vi "AIV.vi"() -> ()   [LabVIEW 2014]
uses:
  <vilib>/Rock Robotics/WPI/SerialPort/WPI_SerialPort.ctl
panel:
  out "all currents (A)":dbl[](array[numeric])
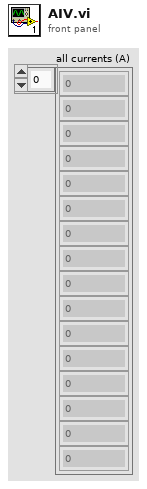
[diagram p1: front panel]
types:
  T1 = typedef "WPI_SerialPort.ctl" = enum16{"Onboard RS-232", "MXP TTL"}
  T2 = typedef "WPI_SerialPortRef.ctl" = cluster{"DevStatus":errorcluster, "Serial Port Name":refnum<visa-resource-name>}
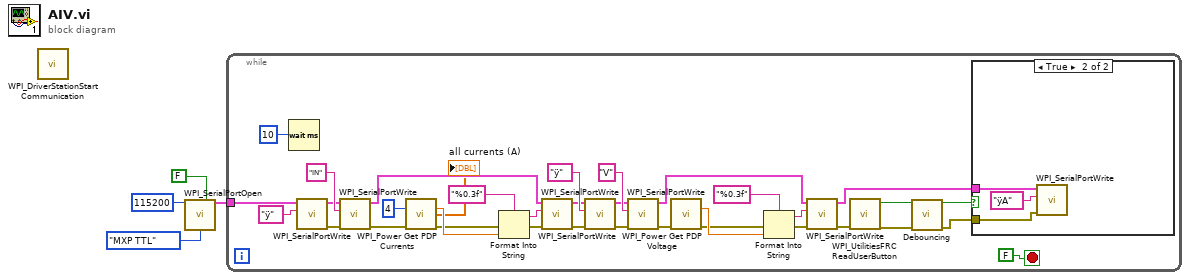
[diagram p0: block diagram]
diagram:
  n1 = call <vilib>:"WPI_DriverStationStart Communication.vi"() -> ()  [unwired: 12 in]
  n2 = call <vilib>:"WPI_SerialPortOpen.vi"("Baud Rate"=u32 115200, "Enable Termination Char? (T)"=FALSE, "Serial Port"=WPI_SerialPort."MXP TTL") -> ("SerialPortRef"=w3:T2)  [unwired: 11 in, 1 out]
  n3 = while {
    tunnel: w3 -> [w36]
    stop <- FALSE stop-if-true
    n4 = Wait (ms)(milliseconds to wait=u32 10) -> ()  [unwired: 1 out]
    n5 = call <vilib>:"WPI_SerialPortWrite.vi"("Buffer"="ÿ", "SerialPortRef"=w36) -> ("error out"=w29:errorcluster, "SerialPortRef"=w30:T2)  [unwired: 7 in, 1 out]
    n6 = call <vilib>:"WPI_SerialPortWrite.vi"("error in (no error)"=w29, "Buffer"="IN", "SerialPortRef"=w30) -> ("error out"=w32:errorcluster, "SerialPortRef"=w25:T2)  [unwired: 6 in, 1 out]
    n7 = call <vilib>:"WPI_Power Get PDP Currents.vi"("PDP Channel"=4, "error in"=w32) -> ("current (A)"=w34:dbl, "all currents (A)"=→"all currents (A)":dbl[], "error out"=w28:errorcluster)  [unwired: 11 in]
    n8 = Format Into String(format string="%0.3f", error in=w28, w34) -> (resulting string=w26:string, error out=w27:errorcluster)  [unwired: 1 in]
    n9 = call <vilib>:"WPI_SerialPortWrite.vi"("error in (no error)"=w27, "Buffer"=w26, "SerialPortRef"=w25) -> ("error out"=w13:errorcluster, "SerialPortRef"=w12:T2)  [unwired: 6 in, 1 out]
    n10 = call <vilib>:"WPI_SerialPortWrite.vi"("error in (no error)"=w13, "Buffer"="ÿ", "SerialPortRef"=w12) -> ("error out"=w18:errorcluster, "SerialPortRef"=w19:T2)  [unwired: 6 in, 1 out]
    n11 = call <vilib>:"WPI_SerialPortWrite.vi"("error in (no error)"=w18, "Buffer"="V", "SerialPortRef"=w19) -> ("error out"=w21:errorcluster, "SerialPortRef"=w14:T2)  [unwired: 6 in, 1 out]
    n12 = call <vilib>:"WPI_Power Get PDP Voltage.vi"("error in"=w21) -> ("voltage (V)"=w22:dbl, "error out"=w17:errorcluster)  [unwired: 13 in]
    n13 = Format Into String(format string="%0.3f", error in=w17, w22) -> (resulting string=w15:string, error out=w16:errorcluster)  [unwired: 1 in]
    n14 = call <vilib>:"WPI_SerialPortWrite.vi"("error in (no error)"=w16, "Buffer"=w15, "SerialPortRef"=w14) -> ("error out"=w11:errorcluster, "SerialPortRef"=w10:T2)  [unwired: 6 in, 1 out]
    n15 = call <vilib>:"WPI_UtilitiesFRC ReadUserButton.vi"("error in"=w11) -> ("error out"=w7:errorcluster, "User Button"=w9:bool)  [unwired: 9 in]
    n16 = call "Debouncing.vi"("error in"=w7, "Input Signal"=w9) -> ("error out"=w6:errorcluster, "Filtered Signal"=w8:bool)  [unwired: 8 in]
    n17 = case shown="True" w8 {
      tunnel: w10 -> [_ w42]
      tunnel: w6 -> [_ w40]
      frame False {
      }
      frame True {
        n18 = call <vilib>:"WPI_SerialPortWrite.vi"("error in (no error)"=w40, "Buffer"="ÿA", "SerialPortRef"=w42) -> ()  [unwired: 6 in, 3 out]
      }
    }
  }
